vi "Read indent.vi"(11 "MsgSerializer in":refnum<class "MsgSerializer.JSON.lvclass">) -> (2 "indent":i32, 3 "MsgSerializer out":refnum<class "MsgSerializer.JSON.lvclass">)   [LabVIEW 2013]
uses:
  MsgSerializer.JSON.lvclass
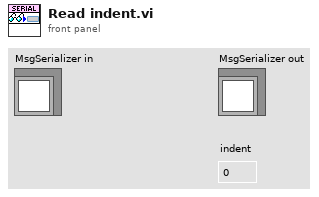
[diagram p1: front panel]
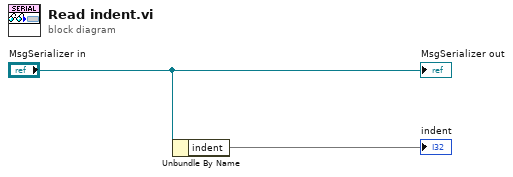
[diagram p0: block diagram]
diagram:
  n1 = Unbundle By Name("MsgSerializer in") -> ("indent"=→"indent")
  "MsgSerializer out" <- "MsgSerializer in"
